vi "Set converted files.vi"(8 "error in (no error)":errorcluster, 10 "converted cxd files":i32, 11 "TomoConversion in":refnum<class "TomoConversion.lvclass">) -> (0 "error out":errorcluster, 3 "TomoConversion out":refnum<class "TomoConversion.lvclass">)   [LabVIEW 2012, in "TomoConversion.lvclass"]
uses:
  TomoConversion.lvclass
  TomoConversion.lvclass/TomoConversion.ctl
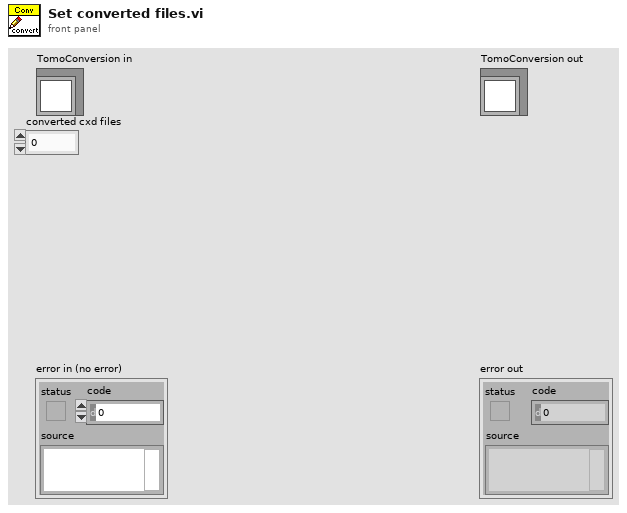
[diagram p1: front panel]
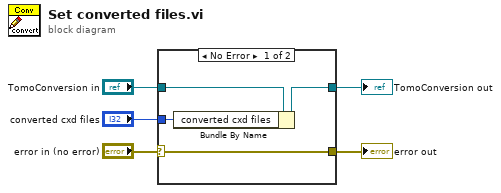
[diagram p0: block diagram]
diagram:
  n1 = case shown="No Error" "error in (no error)" {
    selector: "error in (no error)" -> [w9 w11]
    tunnel: [w9 w11] -> w4
    tunnel: [w7 w10] -> w2
    tunnel: "TomoConversion in" -> [w8 w10]
    tunnel: "converted cxd files" -> [w6 _]
    frame No Error {
      n2 = Bundle By Name(cluster=w8, "converted cxd files"=w6) -> (w7:refnum<class "TomoConversion.lvclass">)
    }
    frame Error {
    }
  }
  "error out" <- w4
  "TomoConversion out" <- w2
